vi "rvc Special Euclidean se2 (vector).vi"(6 "angle unit":u16(ring) items=["radians", "degrees"], 8 "error in (no error)":errorcluster, 11 "Pose":dbl[](array[numeric])) -> (0 "Error Out":errorcluster, 3 "T":dbl[][](array[numeric]))   [LabVIEW 2014]
doc: "This function builds and outputs a 3x3 homogeneous transformation as a 2-D array(T). Inputs are horizontal translation (X), vertical translation (Y), and rotation (theta) in radians. The default value of theta is 0 rad."
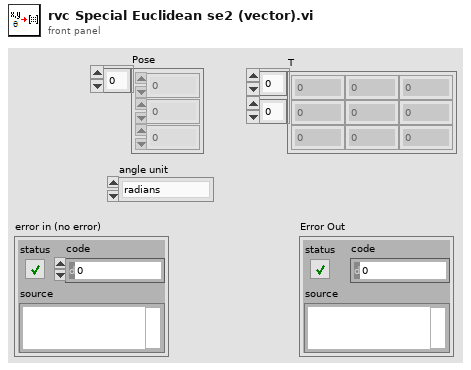
[diagram p1: front panel]
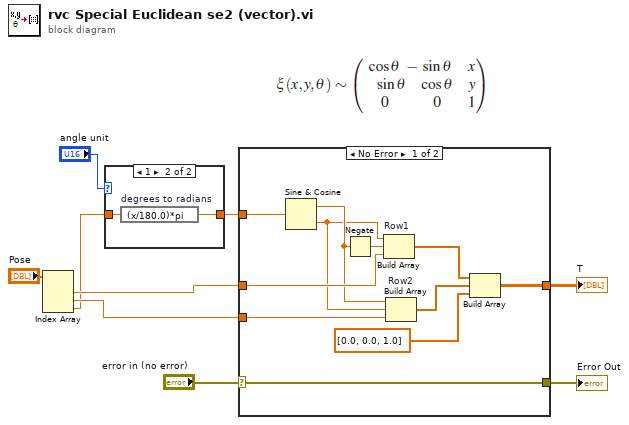
[diagram p0: block diagram]
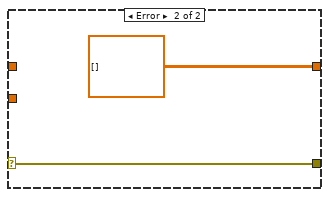
[diagram p3: hidden frame]
diagram:
  n1 = Index Array(array="Pose") -> (element #1=w3:dbl, element #2=w2:dbl, element #3=w1:dbl)  [unwired: 3 in]
  n2 = case shown="1" "angle unit" {
    tunnel: w1 -> [w10 w12]
    tunnel: [w10 w11] -> w6
    frame 0, Default {
    }
    frame 1 {
      n3 = expression code="(x/180.0)*pi" "degrees to radians"(w12) -> (w11:dbl)
    }
  }
  n4 = case shown="No Error" "error in (no error)" {
    selector: "error in (no error)" -> [w23 w24]
    tunnel: [w23 w24] -> w8
    tunnel: w3 -> [w22 _]
    tunnel: w2 -> [w20 _]
    tunnel: w6 -> [w15 _]
    tunnel: [w16 dbl[][] [] ("t")] -> w7
    frame No Error {
      n5 = Sine & Cosine(0:w15) -> (1:w21:dbl, 2:w13:dbl)
      n6 = Negate(x=w21) -> (-x=w14:dbl)
      n7 = Build Array "Row1"(w13, w14, w22) -> (w19:dbl[])
      n8 = Build Array "Row2"(w21, w13, w20) -> (w18:dbl[])
      n9 = Build Array(w19, w18, dbl[] [0.0, 0.0, 1.0] ("appended array")) -> (w16:dbl[][])
    }
    frame Error {
    }
  }
  "Error Out" <- w8
  "T" <- w7
